vi "AllocateSamples.vi"(4 "Samples per Block":i32, 6 "Loop Iteration":i32, 7 "Offset Volt":dbl, 8 "Converted Array In":dbl[](array[numeric]), 10 "Conversion Constant":dbl, 11 "Raw Array In":u8[](array[numeric])) -> (0 "Converted Array out":dbl[](array[numeric]), 3 "Raw Array Out":u8[](array[numeric]), 5 "Missed Samples":i32)   [LabVIEW 2014]
uses:
  Element.ctl
  States.ctl
panel:
  out "Duration":dbl
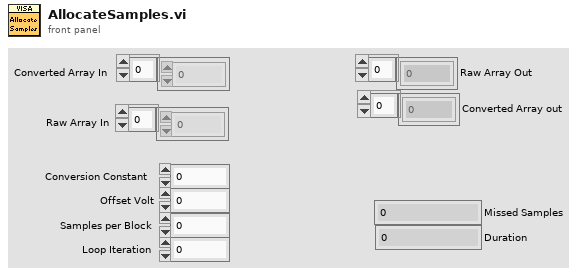
[diagram p1: front panel]
types:
  T1 = enum16{"Acquisition Loop", "VISA Loop", "FFT Loop", "Spectrogram Loop"}
  T2 = typedef "States.ctl" = enum16{"Init", "Flush", "Add"}
  T3 = typedef "Element.ctl" = cluster{"Duration":dbl, "Location":enum16{"Acquisition Loop", "VISA Loop", "FFT Loop", "Spectrogram Loop"}}
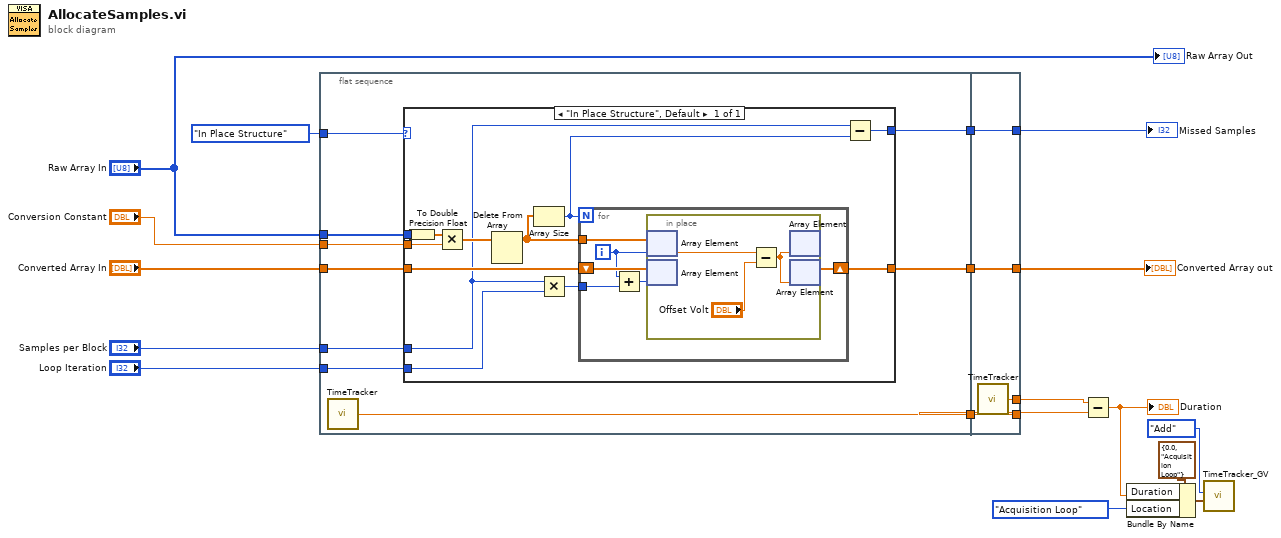
[diagram p0: block diagram]
diagram:
  n1 = flat-sequence {
    tunnel: [w26] -> w11
    tunnel: [w21] -> w10
    tunnel: "Samples per Block" -> [w22]
    tunnel: "Raw Array In" -> [w23]
    tunnel: "Conversion Constant" -> [w24]
    tunnel: "Loop Iteration" -> [w25]
    tunnel: "Converted Array In" -> [w27]
    tunnel: [w20] -> w9
    tunnel: enum16{"In Place Structure", "Array Functions"}."In Place Structure" -> [w19]
    tunnel: [w51] -> w12
    tunnel: [w52] -> w17
    tunnel: w11 -> [w52]
    tunnel: w10 -> [w51]
    tunnel: w9 -> [w50]
    tunnel: [w50] -> w8
    tunnel: [w49] -> w7
    frame #0 {
      n2 = call "TimeTracker.vi"() -> ("Time Out"=w20:dbl)  [unwired: 5 in]
      n3 = case shown="\"In Place Structure\", Default" w19 {
        tunnel: w27 -> [w39]
        tunnel: [w38] -> w26
        tunnel: w25 -> [w37]
        tunnel: w24 -> [w32]
        tunnel: w23 -> [w31]
        tunnel: w22 -> [w29]
        tunnel: [w28] -> w21
        frame "In Place Structure", Default {
          n4 = To Double Precision Float(number=w31) -> (double precision float=w33:dbl[])
          n5 = Multiply(x=w33, y=w32) -> (x*y=w34:dbl[])
          n6 = Delete From Array(array=w34) -> (array with subset deleted=w35:dbl[])  [unwired: 2 in, 1 out]
          n7 = Array Size(array=w35) -> (size(s)=w30:i32)
          n8 = Multiply(x=w29, y=w37) -> (x*y=w36:i32)
          n9 = for {
            N: w30 -> [_]
            shift-right: [w43] -> w38
            shift-left: w39 -> [w44]
            tunnel: w36 -> [w40]
            tunnel: w35 -> [w45]
            i -> [w41]
            n10 = Add(x=w41, y=w40) -> (x+y=w42:i32)
            n11 = in-place {
              n12 = in-place-array #1(w45, w41) -> (w48:dbl)
              n13 = in-place-array #2(w44, w42) -> ()  [unwired: 1 out]
              n14 = Subtract(x=w48, y="Offset Volt") -> (x-y=w47:dbl)
              n15 = in-place-array #1(w47) -> ()  [unwired: 2 out]
              n16 = in-place-array #2(w47) -> (w43:dbl[])  [unwired: 1 out]
            }
          }
          n17 = Subtract(x=w29, y=w30) -> (x-y=w28:i32)
        }
      }
    }
    frame #1 {
      n18 = call "TimeTracker.vi"() -> ("Time Out"=w49:dbl)  [unwired: 5 in]
    }
  }
  n19 = Subtract(x=w7, y=w8) -> (x-y=w3:dbl)
  "Duration" <- w3
  n20 = Bundle By Name(cluster=T3 {"Duration"=0.0, "Location"=enum."Acquisition Loop"} ("Element In"), "Duration"=w3, "Location"=T1."Acquisition Loop") -> (w5:T3)
  n21 = call "TimeTracker_GV.vi"("Action"=States."Add", "Element In"=w5) -> ()  [unwired: 5 in, 1 out]
  "Converted Array out" <- w17
  "Missed Samples" <- w12
  "Raw Array Out" <- "Raw Array In"
